vi "GET MN.vi"(8 "error in (no error)":errorcluster) -> (0 "error out":errorcluster, 2 "PW":string, 3 "MN":string)   [LabVIEW 2022 SP3, in "工况数据上传.lvlib"]
uses:
  <vilib>/registry/registry.llb/Registry RtKey.ctl
  <vilib>/registry/registry.llb/Read Registry Value Simple STR.vi
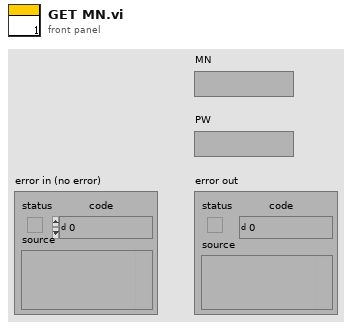
[diagram p1: front panel]
types:
  T1 = typedef "Registry RtKey.ctl" = enum32{"HKEY_CLASSES_ROOT", "HKEY_CURRENT_USER", "HKEY_LOCAL_MACHINE", "HKEY_USERS", "HKEY_PERFORMANCE_DATA", "HKEY_CURRENT_CONFIG", "HKEY_DYN_DATA"}
  T2 = typedef "Registry refnum.ctl" = refnum<k1>
  T3 = cluster{"numValues":i32, "maxValueNameLen":i32, "maxValueDataLen":i32}
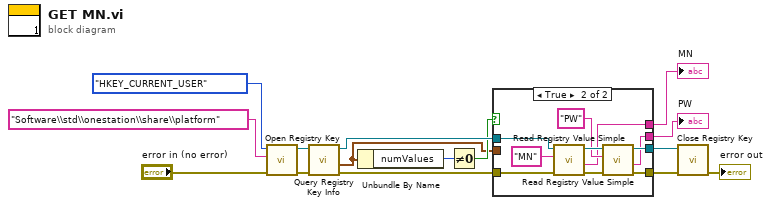
[diagram p0: block diagram]
diagram:
  n1 = call <vilib>:"Open Registry Key.vi"("error in (no error)"="error in (no error)", "subkey"="Software\\std\\onestation\\share\\platform", "root key (HKEY_LOCAL_MACHINE)"=Registry_RtKey."HKEY_CURRENT_USER") -> ("error out"=w10:errorcluster, "refnum out"=w14:T2)  [unwired: 7 in]
  n2 = call <vilib>:"Query Registry Key Info.vi"("error in (no error)"=w10, "refnum"=w14) -> ("error out"=w9:errorcluster, "value info"=w5:T3, "refnum out"=w11:T2)  [unwired: 5 in, 2 out]
  n3 = Unbundle By Name(w5) -> ("numValues"=w8:i32)
  n4 = Not Equal To 0?(x=w8) -> (x != 0?=w7:bool)
  n5 = case shown="True" w7 {
    tunnel: [w17 w23] -> w13
    tunnel: [w16 w21] -> w12
    tunnel: w11 -> [w17 w26]
    tunnel: w9 -> [w16 w25]
    tunnel: w5 -> [_ _]
    tunnel: [_ w19] -> w4
    tunnel: [_ w18] -> w3
    frame False {
    }
    frame True {
      n6 = call-poly <vilib>:"Read Registry Value Simple.vi"("error in (no error)"=w25, "value"="MN", "refnum"=w26) -> ("error out"=w22:errorcluster, "String/Binary data"=w18:string, "refnum out"=w27:T2)  [unwired: 3 in, 1 out]
      n7 = call-poly <vilib>:"Read Registry Value Simple.vi"("error in (no error)"=w22, "value"="PW", "refnum"=w27) -> ("error out"=w21:errorcluster, "String/Binary data"=w19:string, "refnum out"=w23:T2)  [unwired: 3 in, 1 out]
    }
  }
  "PW" <- w4
  "MN" <- w3
  n8 = call <vilib>:"Close Registry Key.vi"("error in (no error)"=w12, "refnum"=w13) -> ("error out"=→"error out":errorcluster)  [unwired: 5 in]
